vi "BinaryStringToValue (Scalar).vi"(1 "String":string) -> (0 "Value":u8)   [LabVIEW 2011, in "UintClass.lvclass"]
uses:
  UintClass.lvclass
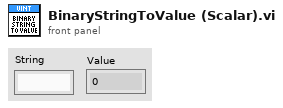
[diagram p1: front panel]
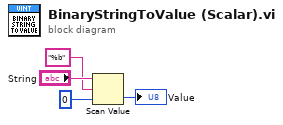
[diagram p0: block diagram]
diagram:
  n1 = Scan Value(string="String", format string="%b", default (0 dbl)=u8 0) -> (value=→"Value":u8)  [unwired: 1 out]
